vi "displayConfigurableElements.vi"(11 "ConfigurationThisComponent in":refnum<class "ConfigurationTestParameters.lvclass">) -> (3 "ConfigurationThisComponent out":refnum<class "ConfigurationTestParameters.lvclass">)   [LabVIEW 2013, in "ConfigurationTestParameters.lvclass"]
uses:
  ConfigurationTestParameters.lvclass
  Configuration/Test Parameters.ctl
  Configuration/CycleProfileConfig.ctl
panel:
  in  "ctrlRefArrayUsrEvnt":refnum<user-event>
  in  "ConfigTab":enum32{"Test Parameters"}(tab)
  in  "Test Parameters":T1={"Number of cycles for complete test"=0, "Cycle profile"={"Force Setpoint"=[], "Pause After"=[]}, "Log Directory"=path "", "Max records per file"=1000, "Comment"=""} {"Max records per file" min=100 max=1000000; "Cycle profile"."Pause After" min=0.0 max=600.0 format="%.1f"; "Cycle profile"."Force Setpoint" min=-888.0 max=888.0 format="%.1f"; "Number of cycles for complete test" min=1}
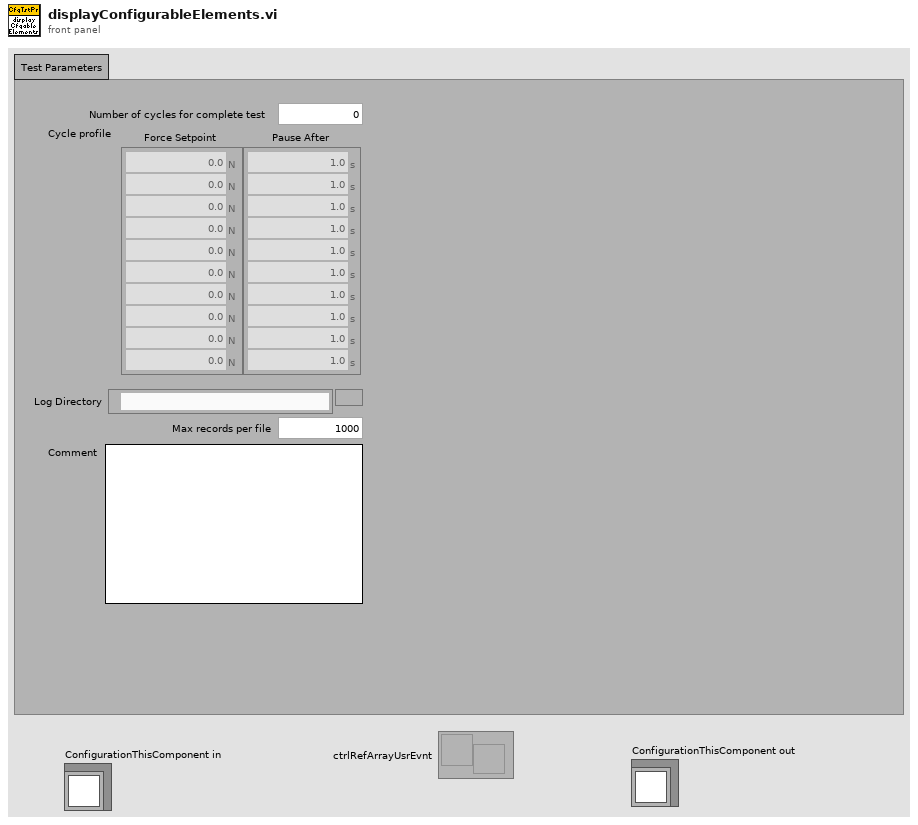
[diagram p1: front panel]
types:
  T1 = typedef "Test Parameters.ctl" = cluster{"Number of cycles for complete test":u32, "Cycle profile":T2, "Log Directory":path, "Max records per file":u32, "Comment":string}
  T2 = typedef "CycleProfileConfig.ctl" = cluster{"Force Setpoint":dbl[unit][], "Pause After":dbl[unit][]}
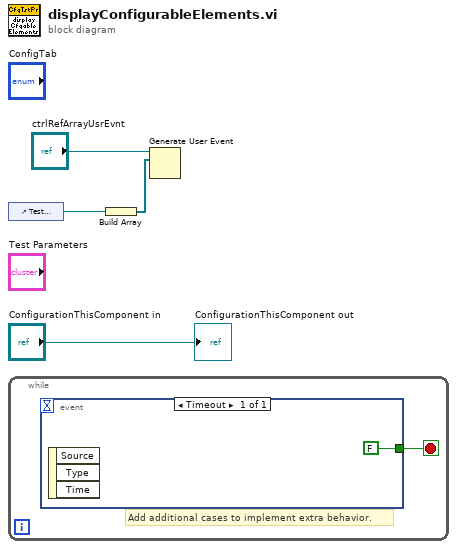
[diagram p0: block diagram]
diagram:
  n1 = control-ref of="Test Parameters"() -> (w2:refnum<vi>)
  n2 = while {
    stop <- w5 stop-if-true
    # "Add additional cases to implement extra behavior."
    n3 = event shown="[0] Timeout" {
      selector: _ -> [_]
      dyn-events: _ -> [_]
      timeout: _ -> [_]
      tunnel: [FALSE] -> w5
      event Timeout {
        n4 = event-data() -> ()  [unwired: 1 in, 3 out]
      }
    }
  }
  n5 = Build Array(w2) -> (w1:refnum<vi>[])
  n6 = Generate User Event(user event="ctrlRefArrayUsrEvnt", event data cluster=w1) -> ()  [unwired: 2 in, 2 out]
  "ConfigurationThisComponent out" <- "ConfigurationThisComponent in"
